vi "Pose Fusion.vi"() -> (0 "pose_out":dbl[](array[numeric]))   [LabVIEW 2025]
uses:
  <vilib>/Rock Robotics/Network Tables/NT Read Float Array.vi
  <vilib>/Rock Robotics/Network Tables/NT Read Number.vi
panel:
  in  "y_tolerance":sgl=0.1
  in  "x_tolerance":sgl=0.1
  out "backcam_pos":sgl[](array[numeric])
  out "frontcam_pos":sgl[](array[numeric])
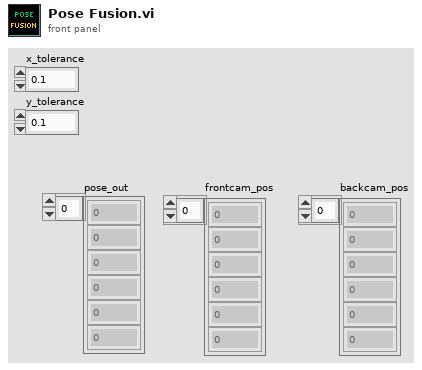
[diagram p1: front panel]
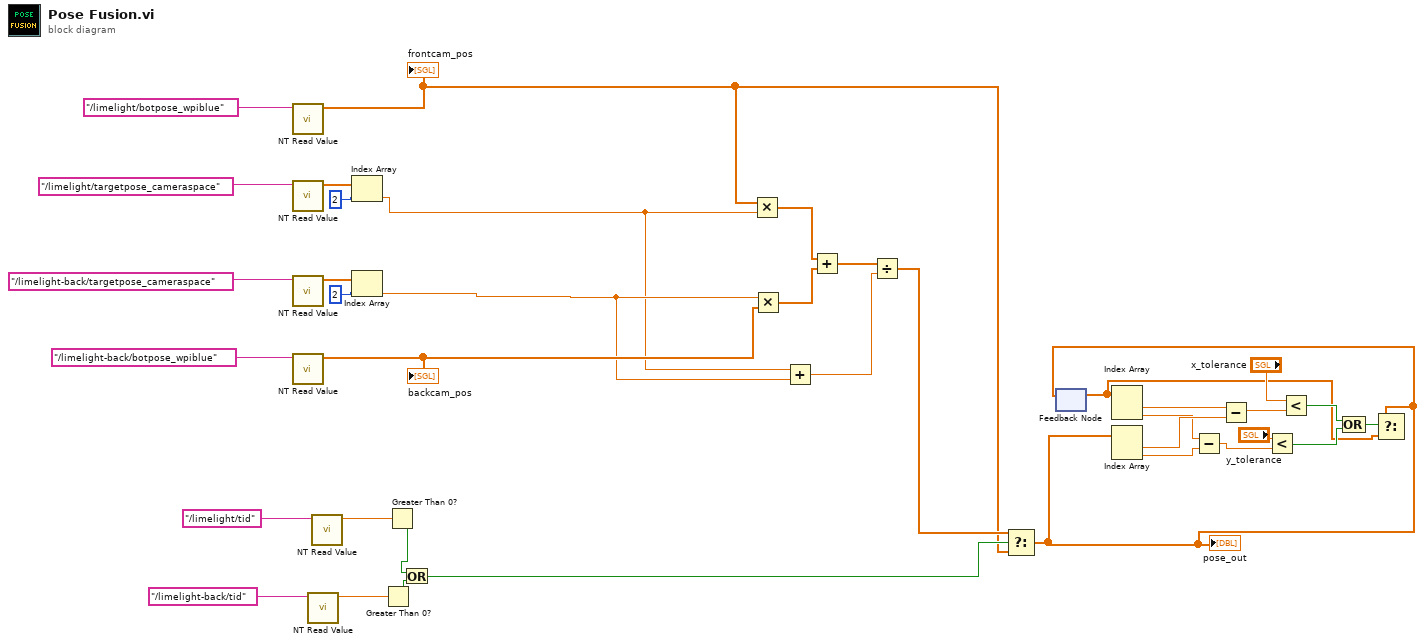
[diagram p0: block diagram]
diagram:
  n1 = call-poly <vilib>:"NT Read Value.vi"("name"="/limelight/botpose_wpiblue") -> ("value"=w16:sgl[])  [unwired: 8 in, 2 out]
  "frontcam_pos" <- w16
  n2 = call-poly <vilib>:"NT Read Value.vi"("name"="/limelight/targetpose_cameraspace") -> ("value"=w29:sgl[])  [unwired: 8 in, 2 out]
  n3 = call-poly <vilib>:"NT Read Value.vi"("name"="/limelight-back/targetpose_cameraspace") -> ("value"=w26:sgl[])  [unwired: 8 in, 2 out]
  n4 = call-poly <vilib>:"NT Read Value.vi"("name"="/limelight-back/botpose_wpiblue") -> ("value"=w37:sgl[])  [unwired: 8 in, 2 out]
  "backcam_pos" <- w37
  n5 = call-poly <vilib>:"NT Read Value.vi"("name"="/limelight-back/tid") -> ("value"=w21:dbl)  [unwired: 8 in, 2 out]
  n6 = call-poly <vilib>:"NT Read Value.vi"("name"="/limelight/tid") -> ("value"=w23:dbl)  [unwired: 8 in, 2 out]
  n7 = Index Array(array=w29, index=2) -> (element=w14:sgl)
  n8 = Index Array(array=w26, index=2) -> (element=w15:sgl)
  n9 = Greater Than 0?(x=w21) -> (x > 0?=w20:bool)
  n10 = Greater Than 0?(x=w23) -> (x > 0?=w19:bool)
  n11 = Or(x=w19, y=w20) -> (x .or. y?=w17:bool)
  n12 = Multiply(x=w16, y=w14) -> (x*y=w36:sgl[])
  n13 = Multiply(x=w15, y=w37) -> (x*y=w35:sgl[])
  n14 = Add(x=w14, y=w15) -> (x+y=w33:sgl)
  n15 = Add(x=w36, y=w35) -> (x+y=w34:sgl[])
  n16 = Divide(x=w34, y=w33) -> (x/y=w18:sgl[])
  n17 = Select(t=w18, s=w17, f=w16) -> (s? t:f=w1:sgl[])
  "pose_out" <- w1
  n18 = feedback-in #1(w1) -> ()
  n19 = feedback #1() -> (w2:sgl[])  [unwired: 1 in]
  n20 = Index Array(array=w2) -> (element #1=w13:sgl, element #2=w11:sgl)  [unwired: 2 in]
  n21 = Index Array(array=w1) -> (element #1=w12:sgl, element #2=w10:sgl)  [unwired: 2 in]
  n22 = Subtract(x=w11, y=w10) -> (x-y=w7:sgl)
  n23 = Subtract(x=w13, y=w12) -> (x-y=w9:sgl)
  n24 = Less?(x="y_tolerance", y=w7) -> (x < y?=w4:bool)
  n25 = Less?(x="x_tolerance", y=w9) -> (x < y?=w5:bool)
  n26 = Compound Arithmetic op=OR(w5, w4) -> (w3:bool)
  n27 = Select(t=w1, s=w3, f=w2) -> ()  [unwired: 1 out]
